vi "Is Concrete Class.vi"(0 "Vector Path Group in":refnum<class "Vector 18GHz Path Group.lvclass">, 11 "error in (no error)":errorcluster) -> (4 "Vector Path Group out":refnum<class "Vector 18GHz Path Group.lvclass">, 6 "Is Concrete Class?":bool=TRUE, 15 "error out":errorcluster)   [LabVIEW 2023, in "RFFixtureCharact.RFPM.lvlib" / "Vector 18GHz Path Group.lvclass"]
uses:
  Vector 18GHz Path Group.lvclass
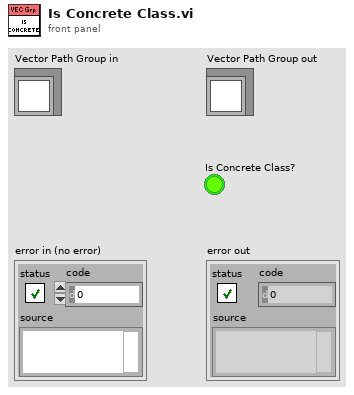
[diagram p1: front panel]
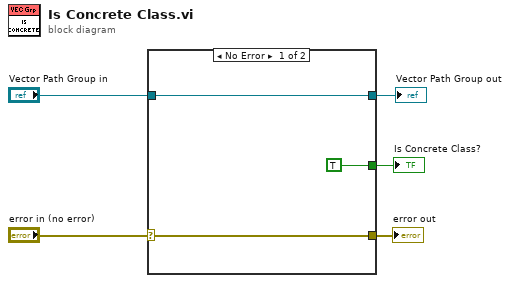
[diagram p0: block diagram]
diagram:
  n1 = case shown="No Error" "error in (no error)" {
    selector: "error in (no error)" -> [w7 w10]
    tunnel: [TRUE ("Is Concrete Class?") _] -> w5
    tunnel: [w7 w10] -> w3
    tunnel: [w6 w9] -> w2
    tunnel: "Vector Path Group in" -> [w6 w9]
    frame No Error {
    }
    frame Error {
    }
  }
  "error out" <- w3
  "Vector Path Group out" <- w2
  "Is Concrete Class?" <- w5
